vi "HIOKI PW3390 Meas NoisePeak.vi"(0 "VISA Resource":refnum<visa-resource-name>, 11 "error in (no error)":errorcluster, 13 "Error Out (F: Off)":bool) -> (4 "VISA Resource out":refnum<visa-resource-name>, 6 "Vf out":dbl[](array[numeric]) format="%.2f", 8 "V out":dbl[](array[numeric]) format="%.2e", 10 "Af out":dbl[](array[numeric]) format="%.2f", 14 "A out":dbl[](array[numeric]) format="%.2e", 15 "error out":errorcluster)   [LabVIEW 2009]
doc: "Reads the frequencies and levels of the top ten highest Noise Measurement voltage and current values.\nThe measurement data's order is fixed."
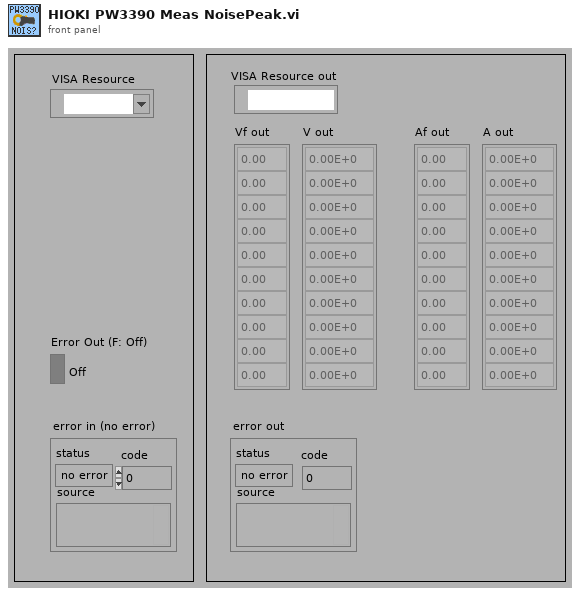
[diagram p1: front panel]
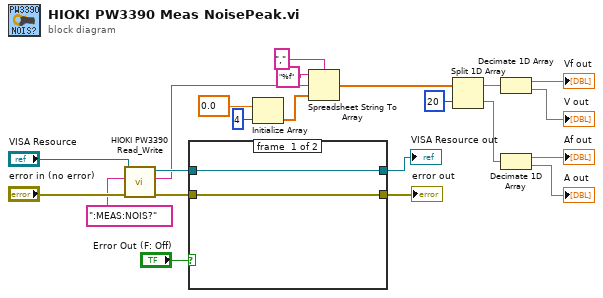
[diagram p0: block diagram]
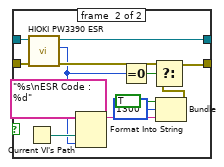
[diagram p2: hidden frame]
diagram:
  n1 = call <instrlib>:"HIOKI PW3390 Read_Write.vi"("error in (no error)"="error in (no error)", "data in"=":MEAS:NOIS?", "VISA Resource"="VISA Resource") -> ("error out"=w9:errorcluster, "data out"=w12:string, "VISA Resource out"=w17:refnum<visa-resource-name>)  [unwired: 6 in]
  n2 = case shown="TRUE" "Error Out (F: Off)" {
    tunnel: w17 -> [w24 w37]
    tunnel: w9 -> [w23 w36]
    tunnel: [w23 w26] -> w21
    tunnel: [w24 w35] -> w1
    frame #0 {
    }
    frame #1 {
      n3 = Current VI's Path() -> (path=w33:path)
      n4 = call <instrlib>:"HIOKI PW3390 ESR.vi"("error in (no error)"=w36, "VISA Resource"=w37) -> ("error out"=w27:errorcluster, "Output Value"=w25:u8, "VISA Resource out"=w35:refnum<visa-resource-name>)  [unwired: 6 in, 1 out]
      n5 = Format Into String(format string="%s\nESR Code : %d", w33, w25) -> (resulting string=w29:string)  [unwired: 2 in, 1 out]
      n6 = Equal To 0?(x=w25) -> (x = 0?=w34:bool)
      n7 = Bundle("status"=TRUE, "code"=1300, w29) -> (w28:cluster{"status":bool, "code":i32, string})  [unwired: 1 in]
      n8 = Select(t=w27, s=w34, f=w28) -> (s? t:f=w26:errorcluster)
    }
  }
  "error out" <- w21
  "VISA Resource out" <- w1
  n9 = Initialize Array(0.0, 4) -> (w11:dbl[])
  n10 = Spreadsheet String To Array(delimiter (Tab)=",", format string="%f", spreadsheet string=w12, array type (2D Dbl)=w11) -> (array=w6:dbl[])
  n11 = Split 1D Array(array=w6, index=20) -> (first subarray=w7:dbl[], second subarray=w5:dbl[])
  n12 = Decimate 1D Array(w7) -> (→"Vf out":dbl[], →"V out":dbl[])
  n13 = Decimate 1D Array(w5) -> (→"Af out":dbl[], →"A out":dbl[])
